vi "FIU line.vi"(8 "error in (no error)":errorcluster, 11 "Node Ptr":T2 format="%.0x") -> (0 "error out":errorcluster)   [LabVIEW 2014, in "SLSC configuration System Explorer.lvlib"]
uses:
  SLSC configuration System Explorer.lvlib
  <vilib>/NI Veristand/Custom Device API/Custom Device Item Ref.ctl
  Shared/FIU Board/Fault State.ctl
  Shared/Constants.vi
  <vilib>/NI Veristand/Custom Device API/Get Item Property (U16).vi
  <vilib>/NI Veristand/Custom Device API/Custom Device API.lvlib
  Shared/SLSC configuration Shared.lvlib
panel:
  out "Fault #":u8=1
  in  "Initial Value":T1
  in  "Header":cluster{"Section Name":string}={"Section Name"="Fault Line Settings"}
  in  "Description":string
  in  "Name":string
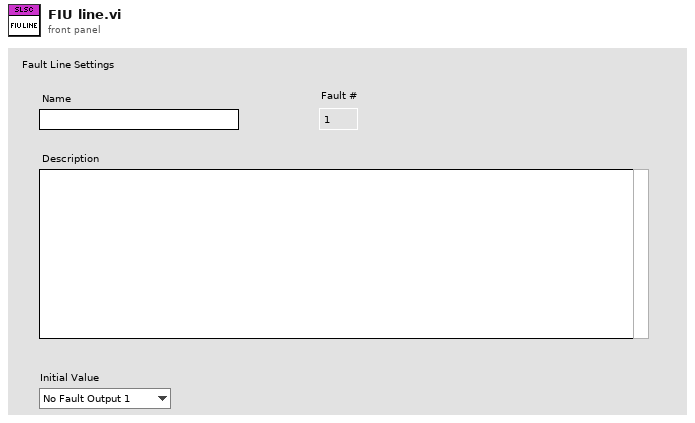
[diagram p1: front panel]
types:
  T1 = typedef "SLSC configuration Shared.lvlib/Fault State.ctl" = enum8{"No Fault Output 1", "Open Circuit 100 Hz", "Ground 100 Hz", "Open Circuit", "Ground", "Fail Rail 1", "Fail Rail 2", "No Fault Output 2"}
  T2 = typedef "Custom Device API.lvlib/Custom Device Item Ref.ctl" = u64
  T3 = typedef "Custom Device API.lvlib/Custom Device Item Info.ctl" = cluster{"Name":string, "Is Channel":bool, "GUID":string, "Is Waveform":bool}
  T4 = typedef "Custom Device API.lvlib/Custom Device Channel.ctl" = cluster{"Type":T5, "Units":string, "Default Value":dbl, "Faultable":bool, "Scalable":bool}
  T5 = typedef "Custom Device API.lvlib/Custom Device Channel Type.ctl" = enum16{"Input", "Output"}
  T6 = typedef "Custom Device API.lvlib/Custom Device Commands.ctl" = enum16{"Default", "Item renamed", "Shutdown", "Dynamic button pressed"}
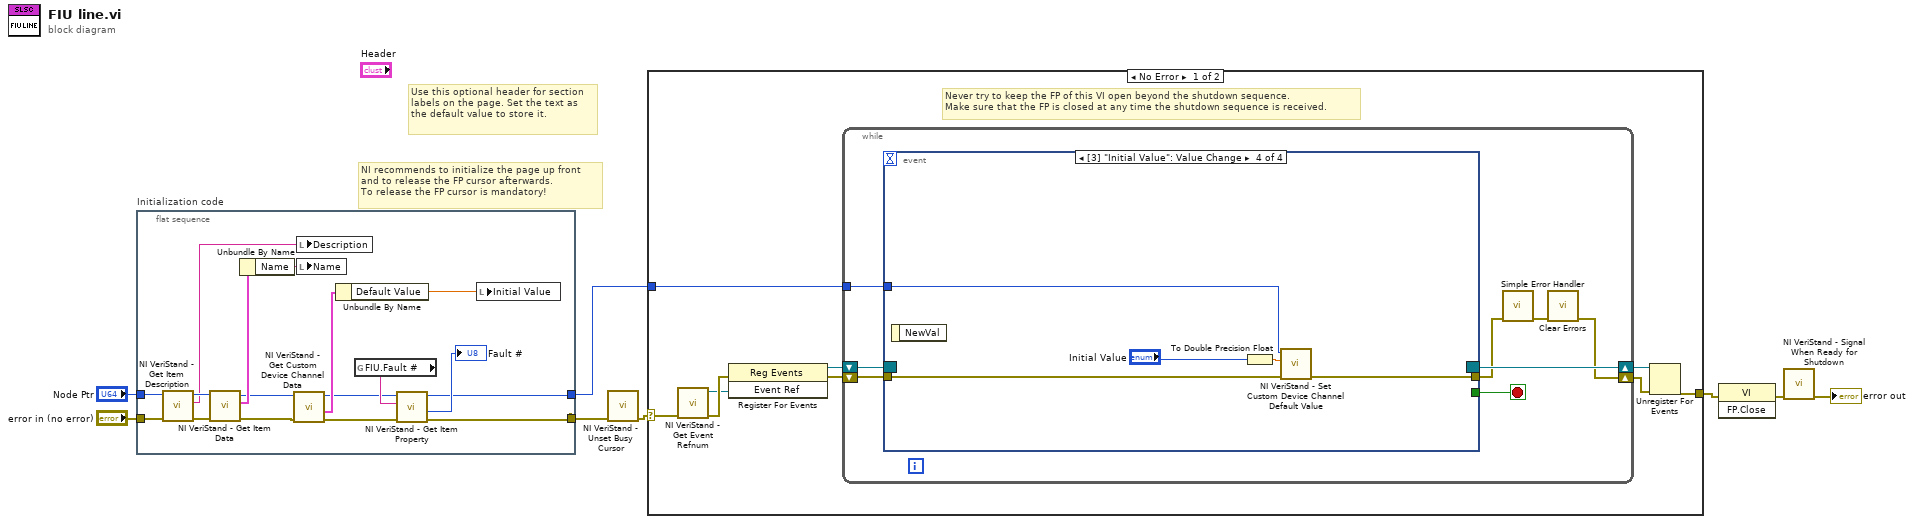
[diagram p0: block diagram]
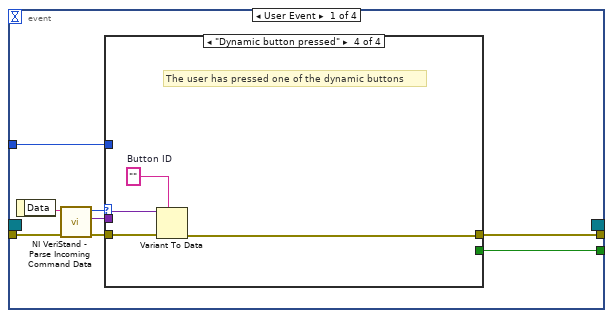
[diagram p2: hidden frame]
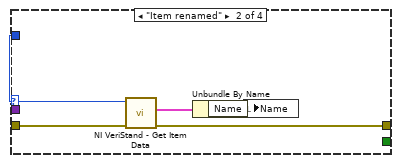
[diagram p4: hidden frame]
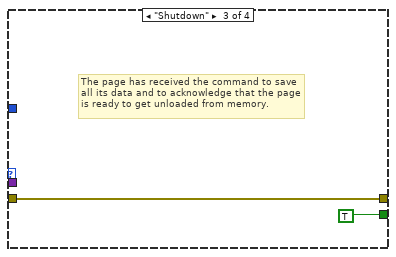
[diagram p5: hidden frame]
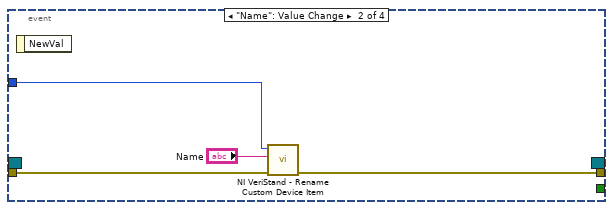
[diagram p6: hidden frame]
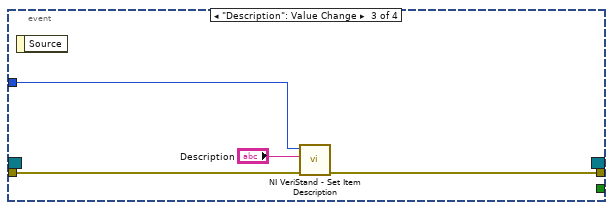
[diagram p7: hidden frame]
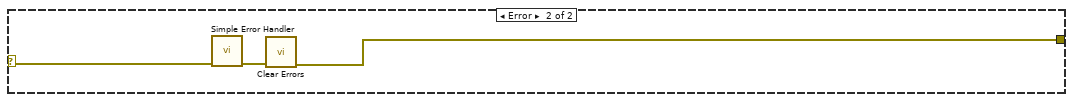
[diagram p8: hidden frame]
diagram:
  # "Use this optional header for section labels on the page. Set the text as the default value to store it."
  # "NI recommends to initialize the page up front\nand to release the FP cursor afterwards.\nTo release the FP cursor is mandatory!"
  n1 = flat-sequence "Initialization code" {
    tunnel: "error in (no error)" -> [w24]
    tunnel: "Node Ptr" -> [w23]
    tunnel: [w10] -> w4
    tunnel: [w9] -> w1
    frame #0 {
      n2 = call <vilib>:"NI VeriStand - Get Item Description.vi"("error in (no error)"=w24, "Item Ref in"=w23) -> ("error out"=w21:errorcluster, "Description"=w22:string, "Item Ref out"=w25:T2)  [unwired: 7 out]
      n3 = call <vilib>:"NI VeriStand - Get Item Data.vi"("error in (no error)"=w21, "Item Ref in"=w25) -> ("error out"=w16:errorcluster, "Item Info"=w20:T3, "Item Ref out"=w17:T2)  [unwired: 7 out]
      n4 = Unbundle By Name(w20) -> ("Name"=w19:string)
      n5 = call <vilib>:"NI VeriStand - Get Custom Device Channel Data.vi"("error in (no error)"=w16, "Channel Ref in"=w17) -> ("error out"=w14:errorcluster, "Channel"=w18:T4, "Channel Ref out"=w11:T2)  [unwired: 4 in, 3 out]
      n6 = local write "Description"(w22) -> ()
      n7 = local write "Name"(w19) -> ()
      n8 = Unbundle By Name(w18) -> ("Default Value"=w15:dbl)
      n9 = global read "Constants.vi" "FIU.Fault #"() -> (w13:string)
      n10 = call-poly <vilib>:"NI VeriStand - Get Item Property.vi"("error in (no error)"=w14, "Property Name"=w13, "Item Ref in"=w11) -> ("error out"=w10:errorcluster, "Value"=→"Fault #":u16, "Item Ref out"=w9:T2)  [unwired: 5 in, 1 out]
      n11 = local write "Initial Value"(w15) -> ()
    }
  }
  n12 = call <vilib>:"NI VeriStand - Unset Busy Cursor.vi"("error in (no error)"=w4) -> ("error out"=w3:errorcluster)  [unwired: 10 out]
  n13 = case shown="No Error" w3 {
    selector: w3 -> [w26 w78]
    tunnel: [w31 w76] -> w8
    tunnel: w1 -> [w27 _]
    frame No Error {
      # "Never try to keep the FP of this VI open beyond the shutdown sequence.\nMake sure that the FP is closed at any time the shutdown sequence is received."
      n14 = call <vilib>:"NI VeriStand - Get Event Refnum.vi"("error in (no error)"=w26) -> ("error out"=w34:errorcluster, "Event Ref"=w30:refnum<user-event>)  [unwired: 9 out]
      n15 = register-events(error in=w34, w30) -> (reference out=w28:refnum<event-registration>, error out=w29:errorcluster)  [unwired: 1 in]
      n16 = while {
        tunnel: w27 -> [w38]
        shift-right: [w35] -> w32
        shift-left: w29 -> [w41]
        shift-right: [w42] -> w33
        shift-left: w28 -> [w40]
        stop <- w39 stop-if-true
        n17 = event shown="[3] \"Initial Value\": Value Change" {
          selector: w40 -> [_ _ _ _]
          dyn-events: [_ _ _ _] -> w42
          timeout: _ -> [_ _ _ _]
          tunnel: w41 -> [w50 w66 w69 w72]
          tunnel: [w46 _ _ _] -> w39
          tunnel: [w45 w65 w68 w71] -> w37
          tunnel: w38 -> [w44 w64 w70 w74]
          event User Event {
            n18 = event-data() -> ("Data"=w49:string)  [unwired: 1 out]
            n19 = call <vilib>:"NI VeriStand - Parse Incoming Command Data.vi"("error in (no error)"=w50, "Incoming data"=w49) -> ("error out"=w48:errorcluster, "Outgoing data"=w43:variant, "Action"=w47:T6)  [unwired: 7 out]
            n20 = case shown="\"Dynamic button pressed\"" w47 {
              tunnel: w48 -> [w51 w56 w57 w62]
              tunnel: [_ _ TRUE _] -> w46
              tunnel: [w51 w53 w57 w59] -> w45
              tunnel: w44 -> [_ w55 _ _]
              tunnel: w43 -> [_ _ _ w61]
              frame "Default", Default {
              }
              frame "Item renamed" {
                n21 = call <vilib>:"NI VeriStand - Get Item Data.vi"("error in (no error)"=w56, "Item Ref in"=w55) -> ("error out"=w53:errorcluster, "Item Info"=w54:T3)  [unwired: 8 out]
                n22 = Unbundle By Name(w54) -> ("Name"=w52:string)
                n23 = local write "Name"(w52) -> ()
              }
              frame "Shutdown" {
                # "The page has received the command to save all its data and to acknowledge that the page is ready to get unloaded from memory."
              }
              frame "Dynamic button pressed" {
                w60 = ""  # Button ID
                # "The user has pressed one of the dynamic buttons"
                n24 = Variant To Data(error in=w62, type=w60, Variant=w61) -> (error out=w59:errorcluster)  [unwired: 1 out]
              }
            }
          }
          event "Name": Value Change {
            n25 = event-data() -> ()  [unwired: 2 out]
            n26 = call <vilib>:"NI VeriStand - Rename Custom Device Item.vi"("error in (no error)"=w66, "New Name"="Name", "Item Ref in"=w64) -> ("error out"=w65:errorcluster)  [unwired: 1 in, 7 out]
          }
          event "Description": Value Change {
            n27 = event-data() -> ()  [unwired: 2 out]
            n28 = call <vilib>:"NI VeriStand - Set Item Description.vi"("error in (no error)"=w69, "Description"="Description", "Item Ref in"=w70) -> ("error out"=w68:errorcluster)  [unwired: 8 out]
          }
          event Value Change {
            n29 = event-data() -> ()  [unwired: 2 out]
            n30 = To Double Precision Float(number="Initial Value") -> (double precision float=w75:dbl)
            n31 = call <vilib>:"NI VeriStand - Set Custom Device Channel Default Value.vi"("error in (no error)"=w72, "Default Value"=w75, "Channel Ref in"=w74) -> ("error out"=w71:errorcluster)  [unwired: 7 in, 1 out]
          }
        }
        n32 = call <vilib>:"Simple Error Handler.vi"("error in (no error)"=w37) -> ("error out"=w36:errorcluster)  [unwired: 1 in, 7 out]
        n33 = call <vilib>:"Clear Errors.vi"("error in (no error)"=w36) -> ("error out"=w35:errorcluster)  [unwired: 1 in, 5 out]
      }
      n34 = Unregister For Events(event registration refnum=w33, error in=w32) -> (error out=w31:errorcluster)
    }
    frame Error {
      n35 = call <vilib>:"Simple Error Handler.vi"("error in (no error)"=w78) -> ("error out"=w77:errorcluster)  [unwired: 1 in, 7 out]
      n36 = call <vilib>:"Clear Errors.vi"("error in (no error)"=w77) -> ("error out"=w76:errorcluster)  [unwired: 1 in, 5 out]
    }
  }
  n37 = invoke class="VI" method="FP.Close"(error in=w8) -> (error out=w7:errorcluster)  [unwired: 2 in, 2 out]
  n38 = call <vilib>:"NI VeriStand - Signal When Ready for Shutdown.vi"("error in (no error)"=w7) -> ("error out"=→"error out":errorcluster)  [unwired: 10 out]
